vi "Configure Modulation(PWM).vi"(0 "VISA resource name":refnum<visa-resource-name>, 1 "Enable OSK Modulation (F: Disable)":bool, 2 "Duty Cycle (20 %)":dbl=20.0, 3 "Pulse Width (0.0002 s)":dbl=0.0002, 5 "Channel (1: Channel 1)":i32(ring)=1 items=["Channel 1"=1, "Channel 2"=2], 7 "PWM Source (0: Internal)":i32(ring) items=["Internal", "External"], 9 "Modulation Waveform (0: Sinusoid)":i32(ring) items=["Sinusoid", "Square", "Triangle", "Ramp", "Nramp", "Noise", "User"], 11 "error in (no error)":errorcluster, 12 "Pulse Hold (1: Duty)":i32(ring)=1 items=["Width", "Duty"], 13 "Frequency (100 Hz)":dbl=100.0) -> (4 "VISA resource name out":refnum<visa-resource-name>, 15 "error out":errorcluster)   [LabVIEW 2012, in "RIGOL DG4000 Series.lvlib"]
doc: "Configures PWM (Pulse Width Modulation) modulation.\n\nNote:\nPWM is only available when Pulse is enabled."
uses:
  <instrlib>/RIGOL DG4000 Series/RIGOL DG4000 Series.lvlib
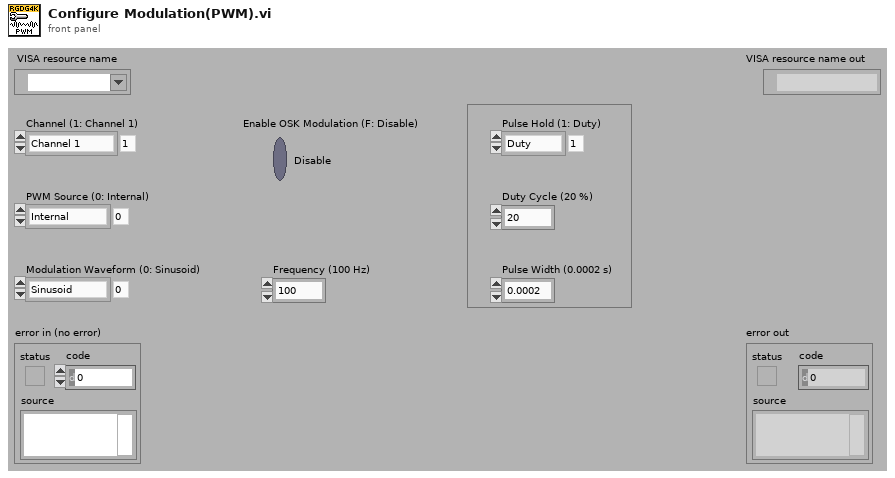
[diagram p1: front panel]
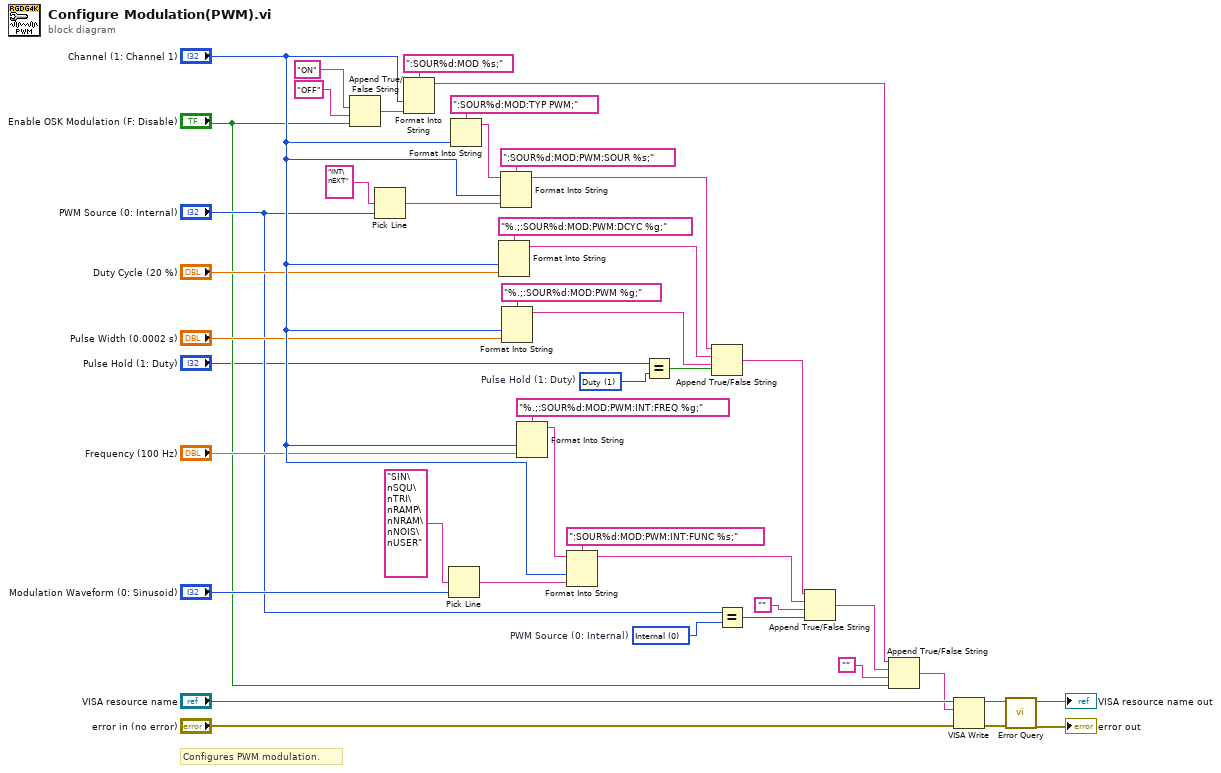
[diagram p0: block diagram]
diagram:
  w3 = 1 items=["Width", "Duty"]  # Pulse Hold (1: Duty)
  w15 = 0 items=["Internal", "External"]  # PWM Source (0: Internal)
  # "Configures PWM modulation."
  n1 = Append True/False String(1:"Enable OSK Modulation (F: Disable)", 2:"OFF", 3:"ON") -> (0:w40:string)  [unwired: 1 out]
  n2 = Pick Line(multi-line string="INT\nEXT", line index="PWM Source (0: Internal)") -> (output string=w35:string)  [unwired: 1 out]
  n3 = Format Into String(format string=":SOUR%d:MOD %s;", "Channel (1: Channel 1)", w40) -> (resulting string=w12:string)  [unwired: 2 in, 1 out]
  n4 = Pick Line(multi-line string="SIN\nSQU\nTRI\nRAMP\nNRAM\nNOIS\nUSER", line index="Modulation Waveform (0: Sinusoid)") -> (output string=w24:string)  [unwired: 1 out]
  n5 = Format Into String(format string=":SOUR%d:MOD:TYP PWM;", "Channel (1: Channel 1)") -> (resulting string=w37:string)  [unwired: 2 in, 1 out]
  n6 = Format Into String(format string="%.;:SOUR%d:MOD:PWM:DCYC %g;", "Channel (1: Channel 1)", "Duty Cycle (20 %)") -> (resulting string=w8:string)  [unwired: 2 in, 1 out]
  n7 = Format Into String(format string=":SOUR%d:MOD:PWM:SOUR %s;", initial string=w37, "Channel (1: Channel 1)", w35) -> (resulting string=w7:string)  [unwired: 1 in, 1 out]
  n8 = Format Into String(format string="%.;:SOUR%d:MOD:PWM %g;", "Channel (1: Channel 1)", "Pulse Width (0.0002 s)") -> (resulting string=w5:string)  [unwired: 2 in, 1 out]
  n9 = Format Into String(format string="%.;:SOUR%d:MOD:PWM:INT:FREQ %g;", "Channel (1: Channel 1)", "Frequency (100 Hz)") -> (resulting string=w26:string)  [unwired: 2 in, 1 out]
  n10 = Format Into String(format string=":SOUR%d:MOD:PWM:INT:FUNC %s;", initial string=w26, "Channel (1: Channel 1)", w24) -> (resulting string=w1:string)  [unwired: 1 in, 1 out]
  n11 = Equal?(x="Pulse Hold (1: Duty)", y=w3) -> (x = y?=w6:bool)
  n12 = Append True/False String(1:w6, 2:w5, 3:w8, 4:w7) -> (0:w2:string)
  n13 = Equal?(x="PWM Source (0: Internal)", y=w15) -> (x = y?=w16:bool)
  n14 = Append True/False String(1:w16, 2:"", 3:w1, 4:w2) -> (0:w11:string)
  n15 = Append True/False String(1:"Enable OSK Modulation (F: Disable)", 2:"", 3:w11, 4:w12) -> (0:w9:string)
  n16 = VISA Write(VISA resource name="VISA resource name", write buffer=w9, error in (no error)="error in (no error)") -> (VISA resource name out=w21:refnum<visa-resource-name>, error out=w20:errorcluster)  [unwired: 1 out]
  n17 = call <instrlib>:"Error Query.vi"("error in (no error)"=w20, "VISA resource name"=w21) -> ("error out"=→"error out":errorcluster, "VISA resource name out"=→"VISA resource name out":refnum<visa-resource-name>)  [unwired: 8 out]
